vi "check Resource Array-Eload.vi"(0 "Resource names":string[](array[string]), 5 "Device current rating":dbl, 9 "Expected current level":dbl, 11 "error in":errorcluster) -> (4 "Single or ganged configuration":bool, 6 "Single/Master resouce name":string, 8 "Slave resource names":string[](array[string]), 10 "Number of devices used":i32, 15 "error out":errorcluster)   [LabVIEW 2021]
doc: "This vi will scan the resource name array and gives out if configuration is single or ganged, along with that it also checks how many eload are required for running the measurement from device current rating."
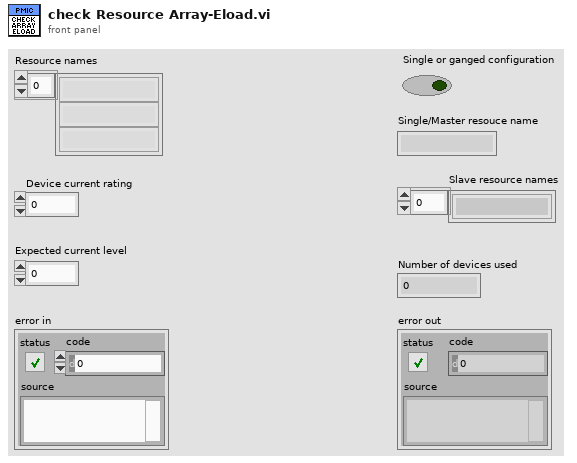
[diagram p1: front panel]
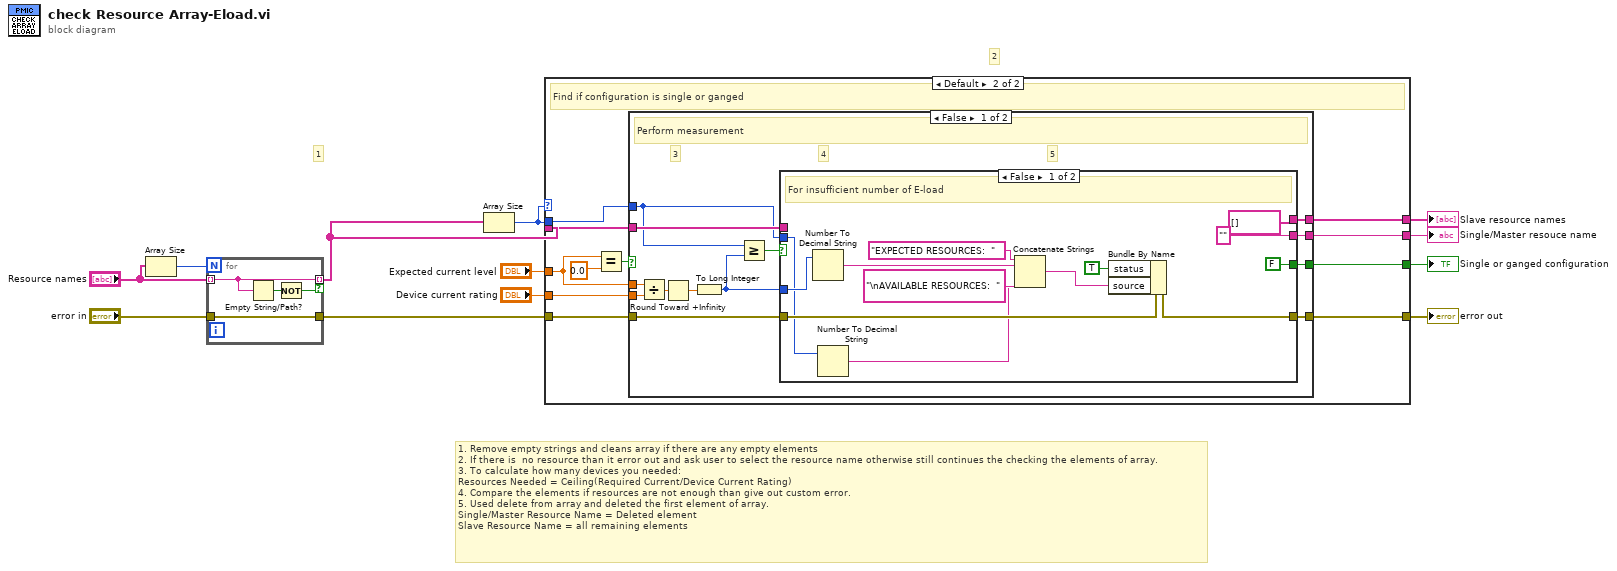
[diagram p0: block diagram]
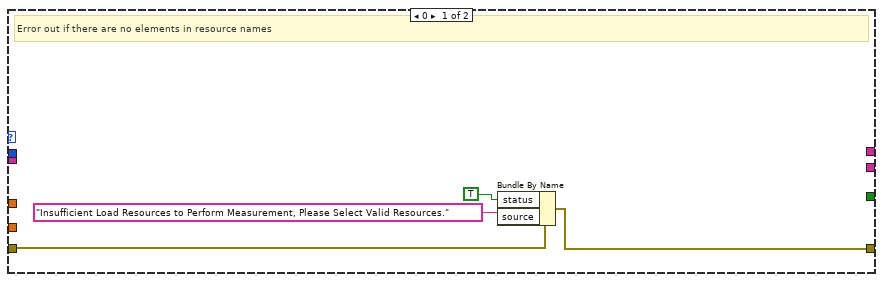
[diagram p2: hidden frame]
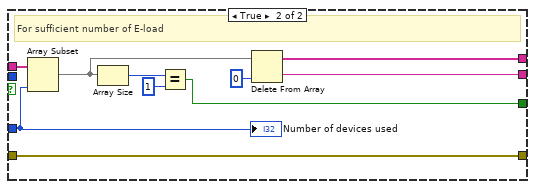
[diagram p3: hidden frame]
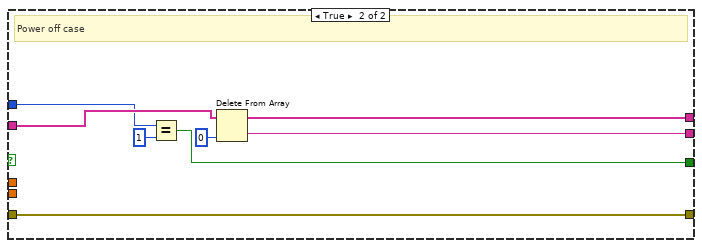
[diagram p4: hidden frame]
diagram:
  # "2"
  # "1"
  # "1. Remove empty strings and cleans array if there are any empty elements\n2. If there is  no resource than it error out and ask user to select the resource name otherwise still continues the checking the elements of array.\n3. To calculate how many devices you needed:\nResources Needed = Ceiling(Required Current/Device Current Rating)\n4. Compare the elements if resources are not enough than give out custom error.\n5. Used delete from array and deleted the first element of array.\nSingle/Master Resource Name = Deleted element\nSlave Resource Name = all remaining elements"
  n1 = Array Size(array="Resource names") -> (size(s)=w9:i32)
  n2 = for {
    N: w9 -> [_]
    tunnel: "Resource names" -> [w15] mode=indexing
    tunnel: "error in" -> [w16]
    tunnel: [w16] -> w8
    tunnel: [w15] -> w7 mode=indexing if=w13
    n3 = Empty String/Path?(string/path=w15) -> (empty?=w14:bool)
    n4 = Not(x=w14) -> (.not. x?=w13:bool)
  }
  n5 = Array Size(array=w7) -> (size(s)=w2:i32)
  n6 = case shown="Default" w2 {
    tunnel: "Device current rating" -> [_ w31]
    tunnel: w8 -> [w18 w30]
    tunnel: w7 -> [_ w29]
    tunnel: "Expected current level" -> [_ w27]
    tunnel: [_ w25] -> w5
    tunnel: [_ w24] -> w4
    tunnel: [_ w23] -> w3
    tunnel: w2 -> [_ w22]
    tunnel: [w17 w21] -> w1
    frame 0 {
      # "Error out if there are no elements in resource names"
      n7 = Bundle By Name(cluster=w18, "status"=TRUE, "source"="Insufficient Load Resources to Perform Measurement, Please Select Valid Resources." ("string")) -> (w17:errorcluster)
    }
    frame Default {
      # "Find if configuration is single or ganged"
      n8 = Equal?(x=w27, y=0.0) -> (x = y?=w28:bool)
      n9 = case shown="False" w28 {
        tunnel: w31 -> [w42 _]
        tunnel: w27 -> [w41 _]
        tunnel: w30 -> [w38 w74]
        tunnel: [w37 w74] -> w21
        tunnel: w29 -> [w36 w71]
        tunnel: [w35 w70] -> w25
        tunnel: [w34 w69] -> w24
        tunnel: [w33 w72] -> w23
        tunnel: w22 -> [w32 w68]
        frame False {
          # "5"
          # "4"
          # "3"
          # "Perform measurement"
          n10 = Divide(x=w41, y=w42) -> (x/y=w44:dbl)
          n11 = Round Toward +Infinity(x=w44) -> (ceil(x): smallest int >= x=w43:dbl)
          n12 = To Long Integer(number=w43) -> (32bit integer=w40:i32)
          n13 = Greater Or Equal?(x=w32, y=w40) -> (x >= y?=w39:bool)
          n14 = case shown="False" w39 {
            tunnel: w36 -> [_ w63]
            tunnel: w40 -> [w49 w62]
            tunnel: w38 -> [w56 w61]
            tunnel: [w57 w61] -> w37
            tunnel: w32 -> [w48 _]
            tunnel: [string[] [] w60] -> w35
            tunnel: ["" ("String") w59] -> w34
            tunnel: [FALSE w58] -> w33
            frame False {
              # "For insufficient number of E-load"
              n15 = Number To Decimal String(number=w49) -> (decimal integer string=w52:string)  [unwired: 1 in]
              n16 = Number To Decimal String(number=w48) -> (decimal integer string=w51:string)  [unwired: 1 in]
              n17 = Concatenate Strings("EXPECTED RESOURCES:  " ("string"), w52, "\nAVAILABLE RESOURCES:  " ("string"), w51) -> (w55:string)
              n18 = Bundle By Name(cluster=w56, "status"=TRUE, "source"=w55) -> (w57:errorcluster)
            }
            frame True {
              # "For sufficient number of E-load"
              n19 = Array Subset(array=w63, length=w62) -> (w65:string[])  [unwired: 1 in]
              n20 = Array Size(array=w65) -> (size(s)=w67:i32)
              n21 = Equal?(x=w67, y=1) -> (x = y?=w58:bool)
              n22 = Delete From Array(array=w65, index=0) -> (deleted portion=w59:string, array with subset deleted=w60:string[])  [unwired: 1 in]
              "Number of devices used" <- w62
            }
          }
        }
        frame True {
          # "Power off case"
          n23 = Equal?(x=w68, y=1) -> (x = y?=w72:bool)
          n24 = Delete From Array(array=w71, index=0) -> (deleted portion=w69:string, array with subset deleted=w70:string[])  [unwired: 1 in]
        }
      }
    }
  }
  "Single/Master resouce name" <- w4
  "Slave resource names" <- w5
  "Single or ganged configuration" <- w3
  "error out" <- w1
